vi "Write Key String.vi"(7 "rel_path":string, 8 "error in (no error)":errorcluster, 9 "value":string, 10 "key":string, 11 "section":string) -> (0 "error out":errorcluster)   [LabVIEW 2016]
uses:
  <vilib>/Utility/config.llb/Write Key (String).vi
  <vilib>/Utility/config.llb/NI_LVConfig.lvlib
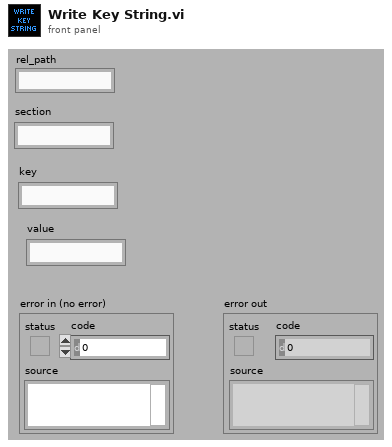
[diagram p1: front panel]
types:
  T1 = enum32{"invalid app kind", "Development System", "Run Time System", "Student Edition", "Embedded LabVIEW", "Evaluation", "Custom"}
  T2 = typedef "NI_LVConfig.lvlib/Config Data RefNum.ctl" = refnum<k1>
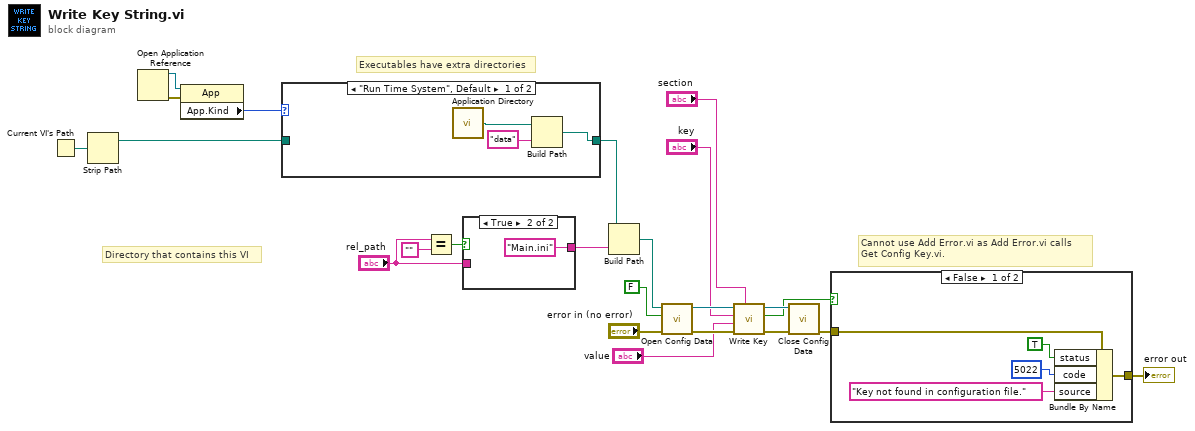
[diagram p0: block diagram]
diagram:
  # "Executables have extra directories"
  # "Directory that contains this VI"
  # "Cannot use Add Error.vi as Add Error.vi calls\nGet Config Key.vi."
  n1 = Current VI's Path() -> (path=w7:path)
  n2 = Strip Path(path=w7) -> (stripped path=w2:path)  [unwired: 1 out]
  n3 = Open Application Reference() -> (0:w5:errorcluster, 3:w6:refnum<vi>)  [unwired: 4 in]
  n4 = property class="App"(reference=w6, error in=w5) -> ("App.Kind"=w3:T1)  [unwired: 2 out]
  n5 = case shown="\"Run Time System\", Default" w3 {
    tunnel: w2 -> [_ w27]
    tunnel: [w26 w27] -> w1
    frame "Run Time System", Default {
      n6 = call <vilib>:"Application Directory.vi"() -> ("Application Directory"=w24:path)
      n7 = Build Path(base path=w24, name or relative path="data") -> (appended path=w26:path)
    }
    frame "Development System" {
    }
  }
  n8 = Equal?(x="rel_path", y="") -> (x = y?=w13:bool)
  n9 = case shown="True" w13 {
    tunnel: [w28 "Main.ini" ("name or relative path")] -> w11
    tunnel: "rel_path" -> [w28 _]
    frame False {
    }
    frame True {
    }
  }
  n10 = Build Path(base path=w1, name or relative path=w11) -> (appended path=w23:path)
  n11 = call <vilib>:"Open Config Data.vi"("error in (no error)"="error in (no error)", "create file if necessary (T)"=FALSE, "configuration file path"=w23) -> ("error out"=w18:errorcluster, "refnum"=w21:T2)  [unwired: 6 in, 1 out]
  n12 = call-poly <vilib>:"Write Key.vi"("section"="section", "error in (no error)"=w18, "value"="value", "key"="key", "refnum"=w21) -> ("error out"=w17:errorcluster, "found?"=w8:bool, "refnum out"=w16:T2)  [unwired: 4 in]
  n13 = call <vilib>:"Close Config Data.vi"("error in (no error)"=w17, "refnum"=w16) -> ("error out"=w9:errorcluster)  [unwired: 8 in, 1 out]
  n14 = case shown="False" w8 {
    tunnel: [w32 w35] -> w10
    tunnel: w9 -> [w30 w35]
    frame False {
      n15 = Bundle By Name(cluster=w30, "status"=TRUE, "code"=5022, "source"="Key not found in configuration file.") -> (w32:errorcluster)
    }
    frame True {
    }
  }
  "error out" <- w10
